vi "FieldOrientedTransform.vi"(7 "Robot Heading (deg)":dbl, 8 "Joystick Y":dbl, 11 "Joystick X":dbl) -> (0 "Joystick Y'":dbl, 3 "Joystick X'":dbl)   [LabVIEW 2019]
doc: "Transforms X and Y joystick axes based on the robot's current orientation, allowing a swerve robot to be controlled in the field-oriented reference frame. The code is primarily based on code included in the FRC WPI Library."
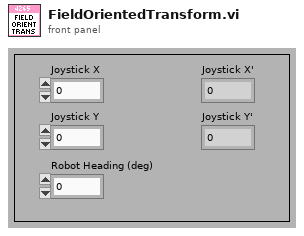
[diagram p1: front panel]
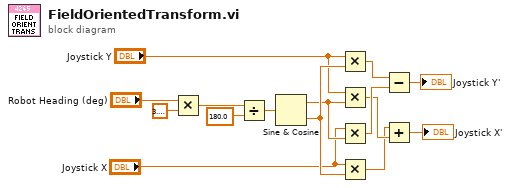
[diagram p0: block diagram]
diagram:
  n1 = Multiply(x="Robot Heading (deg)", y=3.141592653589793) -> (x*y=w5:dbl)
  n2 = Divide(x=w5, y=180.0) -> (x/y=w7:dbl)
  n3 = Sine & Cosine(0:w7) -> (1:w11:dbl, 2:w12:dbl)
  n4 = Multiply(x="Joystick Y", y=w12) -> (x*y=w13:dbl)
  n5 = Multiply(x="Joystick Y", y=w11) -> (x*y=w9:dbl)
  n6 = Multiply(x="Joystick X", y=w11) -> (x*y=w14:dbl)
  n7 = Multiply(x="Joystick X", y=w12) -> (x*y=w8:dbl)
  n8 = Subtract(x=w13, y=w14) -> (x-y=→"Joystick Y'":dbl)
  n9 = Add(x=w8, y=w9) -> (x+y=→"Joystick X'":dbl)
